vi "test matrix_mul.vi"() -> ()   [LabVIEW 2020]
uses:
  <vilib>/rvi/linearAlgebra/MatrixMultiply/simVIs/SubVI/nifxpla_MatrixMultiply_SimMatrixSizes.vi
  <vilib>/rvi/linearAlgebra/MatrixMultiply/simVIs/SubVI/nifxpla_MatrixMultiply_Sim4WireAdapterElement.vi
  <vilib>/rvi/linearAlgebra/MatrixMultiply/simVIs/SubVI/nifxpla_MatrixMultiply_SimFrameHandShake.vi
  <vilib>/rvi/linearAlgebra/MatrixMultiply/simVIs/SubVI/nifxpla_MatrixMultiply_SimScalarDataBuffer.vi
  <vilib>/rvi/linearAlgebra/MatrixMultiply/simVIs/SubVI/nifxpla_MatrixMultiply_SimNestedIndex.vi
  <vilib>/rvi/ClientSDK/Core/DevComputerLib/Private/Multiply(dfxp64).vi
  <vilib>/rvi/ClientSDK/Core/DevComputerLib/Private/Dfxp128ToDfxp256.vi
  <vilib>/rvi/ClientSDK/Core/DevComputerLib/Private/Add(dfxp256).vi
  <vilib>/rvi/ClientSDK/Core/DevComputerLib/Private/Subtract(dfxp256).vi
  <vilib>/rvi/ClientSDK/Core/DevComputerLib/Private/ToDfxp64(dfxp256).vi
  <vilib>/rvi/linearAlgebra/MatrixMultiply/XNode/nifxpla_MatrixMultiply.xnode
  <vilib>/rvi/linearAlgebra/MatrixMultiply/simVIs/nifxpla_MatrixMultiply_SimTemplateEinEout.vi
panel:
  out "ci":fxp<+/-,34,4>
  out "cr":fxp<+/-,34,4>
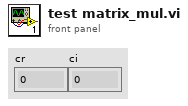
[diagram p1: front panel]
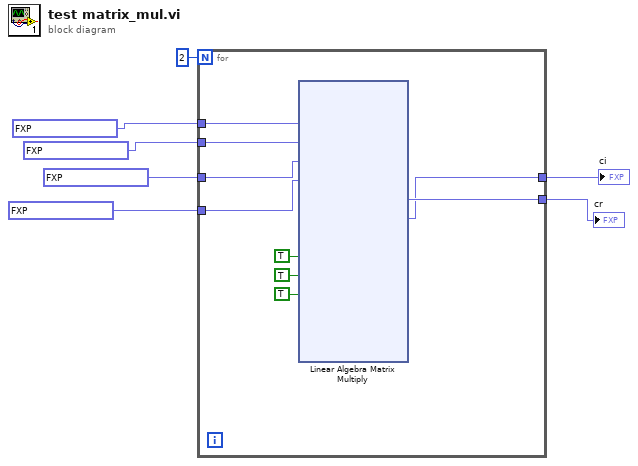
[diagram p0: block diagram]
diagram:
  n1 = for {
    N: 2 -> [_]
    tunnel: fxp<+/-,16,1> 0.999969482421875 ("ar") -> [w16]
    tunnel: fxp<+/-,16,1> 0.999969482421875 ("ai") -> [w15]
    tunnel: fxp<+/-,16,1> 0.999969482421875 ("br") -> [w14]
    tunnel: fxp<+/-,16,1> 0.999969482421875 ("bi") -> [w13]
    tunnel: [w9] -> w3
    tunnel: [w8] -> w2
    n2 = xnode "Linear Algebra Matrix Multiply"("ar"=w16, "ai"=w15, "br"=w14, "bi"=w13, "a valid"=TRUE, "b valid"=TRUE, "ready for output (T)"=TRUE) -> ("cr"=w9:fxp<+/-,34,4>, "ci"=w8:fxp<+/-,34,4>)  [unwired: 4 out]
  }
  "cr" <- w3
  "ci" <- w2
